vi "Save JSON File.vi"(8 "error in (no error)":errorcluster, 10 "Data":variant, 11 "Control Experiment":refnum<class "Control Experiment.lvclass">) -> (0 "error out":errorcluster, 2 "JSON String":string, 3 "Control Experiment out":refnum<class "Control Experiment.lvclass">)   [LabVIEW 2016, in "Control Experiment.lvclass"]
uses:
  Control Experiment.lvclass
  <vilib>/addons/_JKI.lib/Serialization/JSON/JKI JSON Serialization.lvlib
  C:/Program Files (x86)/National Instruments/LabVIEW 2016/user.lib/LevyLab/Levylab Instruments/SMOs/Instrument/Instrument.lvclass
  C:/Program Files (x86)/National Instruments/LabVIEW 2016/vi.lib/JKI/JKI SMO/SMO/SMO.lvclass
  Control Experiment SM/Control Experiment SM.lvclass
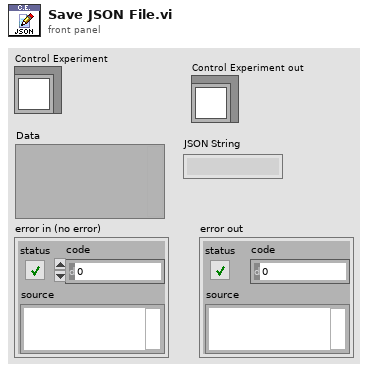
[diagram p1: front panel]
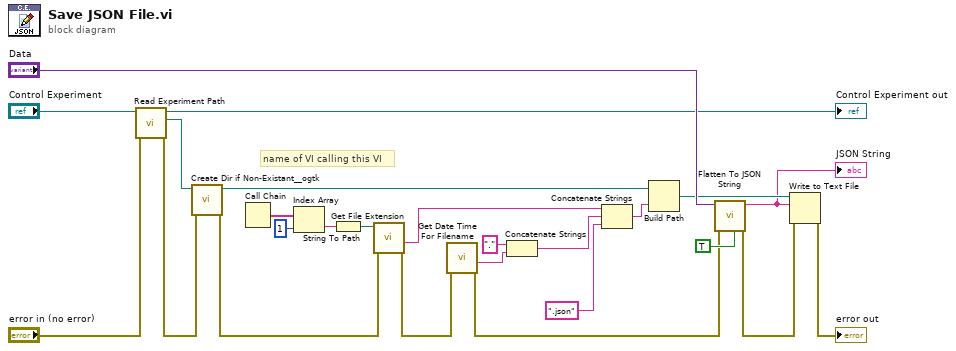
[diagram p0: block diagram]
diagram:
  # "name of VI calling this VI"
  n1 = call "Read Experiment Path.vi"("error in (no error)"="error in (no error)", "Control Experiment in"="Control Experiment") -> ("error out"=w17:errorcluster, "Experiment Path"=w13:path, "Control Experiment out"=→"Control Experiment out":refnum<class "Control Experiment SM.lvclass">)  [unwired: 7 in]
  n2 = call <userlib>:"Create Dir if Non-Existant__ogtk.vi"("error in (no error)"=w17, "Directory Path"=w13) -> ("error out"=w9:errorcluster, "dup Directory Path"=w4:path)  [unwired: 7 in, 1 out]
  n3 = Call Chain() -> (call chain=w22:string[])
  n4 = Index Array(array=w22, index=1) -> (element=w23:string)
  n5 = String To Path(string=w23) -> (path=w25:path)
  n6 = call <vilib>:"Get File Extension.vi"("error in (no error)"=w9, "file"=w25) -> ("error out"=w10:errorcluster, "filename without extension"=w8:string)  [unwired: 5 in, 3 out]
  n7 = call "Get Date Time For Filename.vi"("error in (no error)"=w10) -> ("error out"=w1:errorcluster, "date-time string"=w6:string)  [unwired: 8 in, 1 out]
  n8 = Concatenate Strings("." ("string"), w6) -> (w5:string)
  n9 = Concatenate Strings(w8, w5, ".json" ("string")) -> (w20:string)
  n10 = Build Path(base path=w4, name or relative path=w20) -> (appended path=w12:path)
  n11 = call <vilib>:"Flatten To JSON String.vi"("Enums As String (F)"=TRUE, "error in (no error)"=w1, "Variant"="Data") -> ("error out"=w16:errorcluster, "JSON String"=w2:string)  [unwired: 7 in]
  "JSON String" <- w2
  n12 = Write to Text File(file (use dialog)=w12, text=w2, error in=w16) -> (error out=→"error out":errorcluster)  [unwired: 1 in, 2 out]
